vi "RPS Tools.vi"() -> ()   [LabVIEW 2020]
uses:
  Support/Curve fitting data.ctl
panel:
  out "IR Película 2":dbl format="%#.4g"
  out "ángulo B valor medio":dbl
  out "otros ángulos cero":dbl[](array[numeric])
  in  "Stop":bool
  in  "Tab Control":T1(tab)
  in  "Extinction Coefficients TC":dbl[](array[slide]) caption="Extinction Coefficients" step=0.01 scale=-5.0..5.0
  in  "Thicknesses (angstroms) TC":dbl[](array[slide]) caption="Thicknesses (angstroms)" step=5.0 scale=0.0..1000.0 scale format="%#.6g"
  in  "Refractive Indexes TC":dbl[](array[slide]) caption="Refractive Indexes" step=0.01 scale=1.0..5.0 scale format="%#.6g"
  out "q R theoretical TC":dbl caption="qR theoretical" format="%#.5g"
  in  "No.  Layers TC":u32=1 caption="No.  Layers"
  in  "q maximum TC":dbl=89.0 caption="q maximum"
  in  "q minimum TC":dbl=30.0 caption="q minimum"
  in  "l(angstroms) TC":dbl=6328.0 caption="l(angstroms)"
  in  "Resolution TC":dbl=1000.0 caption="Resolution"
  out "SPR Curve":cluster{"EJE X":dbl[], "EJE Y TEÓRICO":dbl[]}(graph)
  in  "No. Layers CF":u32=1 caption="No. Layers"
  in  "l(angstroms) CF":dbl=6328.0 caption="l(angstroms)"
  in  "Losses CF":dbl(slide)=0.9 caption="Losses" step=0.001 scale=0.0..1.0 scale format="%#.6g"
  in  "Error CF":dbl(slide) caption="Error" step=0.01 scale=-5.0..5.0
  in  "Refractive Indexes CF":dbl[](array[slide]) caption="Refractive Indexes" step=0.001 scale=1.0..5.0 scale format="%#.6g"
  in  "Extinction Coefficients CF":dbl[](array[slide]) caption="Extinction Coefficients" step=0.001 scale=-5.0..5.0 scale format="%#.6g"
  in  "Open File":path
  in  "Thicknesses (angstroms) CF":dbl[](array[slide]) caption="Thicknesses (angstroms)" scale=0.0..1000.0 scale format="%#.6g"
  out "CURVE FITTING":T2(graph)
  in  "Load curve":bool
  out "SPR Curve":cluster{"EJE X":dbl[], dbl[]}(graph)
  in  "q Final ECA":dbl caption="q Final"
  in  "q Starting ECA":dbl caption="q Starting"
  in  "Open File ECA":path caption="Open File"
  in  "Realizar Análisis ECA":bool caption="Realizar Análisis"
  out "qR ECA":dbl caption="qR"
  out "Curve width ECA":dbl caption="Curve width" format="%#.3g"
  out "q  Middle ECA":dbl caption="q  Middle"
  out "Minimun Intensity ECA":dbl caption="Minimun Intensity"
  out "Maximum Intensity ECA":dbl caption="Maximum Intensity"
  in  "Calcular ERROR":bool
  out "RI +error BRW":dbl caption="RI +error" format="%#_4g"
  out "qB +error BRW":dbl caption="qB +error"
  in  "Error (degrees) BRW":dbl caption="Error (degrees)"
  out "Refractive Index BRW":dbl caption="Refractive Index" format="%#.4g"
  out "qB BRW":dbl caption="qB"
  in  "Calcular":bool
  in  "q Final BRW":dbl caption="q Final"
  in  "q Starting BRW":dbl caption="q Starting"
  in  "Open File BRW":path caption="Open File"
  out "Curve":cluster{dbl[], dbl[]}(graph)
  out "Curves":cluster{dbl[], dbl[]}[](graph)
  in  "q Final AB":dbl caption="q Final"
  in  "q Starting AB":dbl caption="q Starting"
  in  "Open Film File AB":path caption="Open Film File"
  in  "Open Substrate File AB":path caption="Open Substrate File"
  in  "OK Button":bool
  out "Film RI AB":dbl caption="Film RI" format="%#.4g"
  out "Substrate RI AB":dbl caption="Substrate RI" format="%#.4g"
  out "Substrate qB AB":dbl caption="Substrate qB"
  out "Film qB AB":dbl caption="Film qB"
  in  "calcular error":bool
  in  "Error (degrees) AB":dbl caption="Error (degrees)"
  out "Film qB +error AB":dbl caption="Film qB +error"
  out "Film RI +error AB":dbl caption="Film RI +error" format="%#.4g"
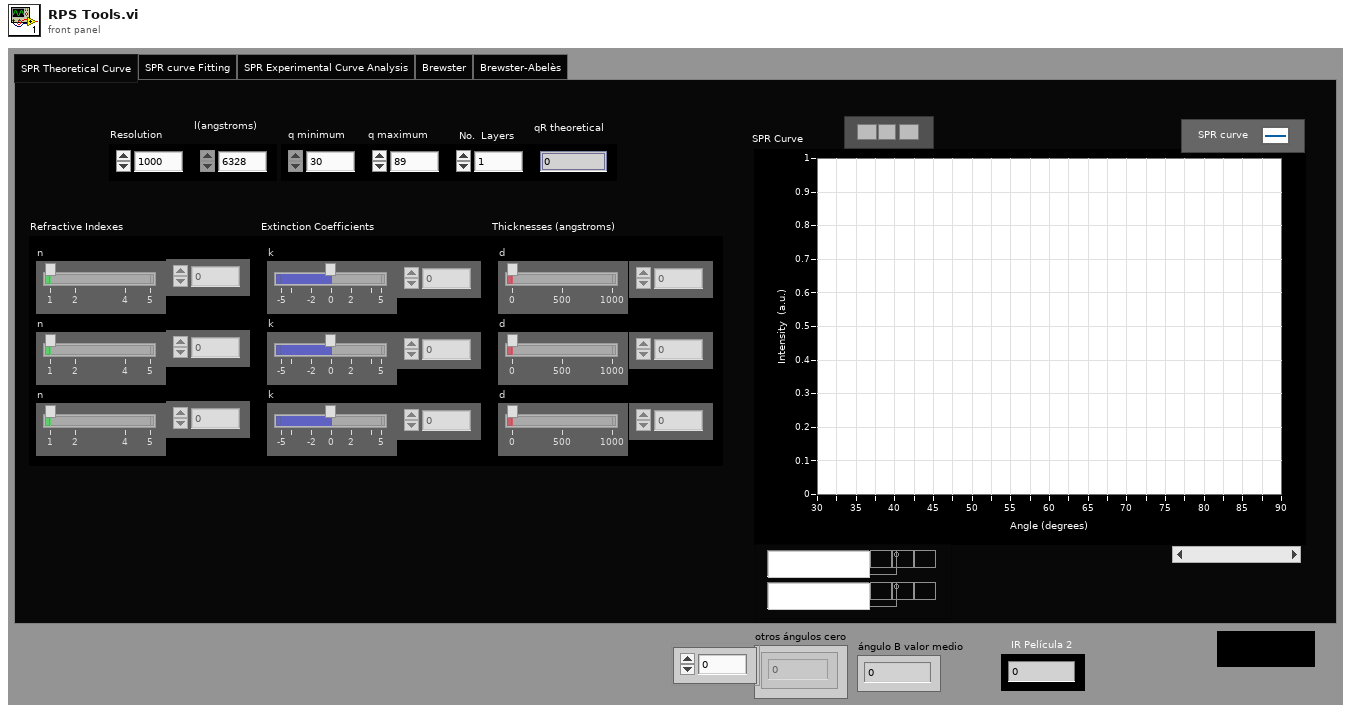
[diagram p1: front panel]
types:
  T1 = enum32{"SPR Theoretical Curve", "SPR curve Fitting", "SPR Experimental Curve Analysis", "Brewster", "Brewster-Abelès"}
  T2 = cluster{"EJE X":dbl[], "EJE Y NORMALIZADO":dbl[]}[]
  T3 = typedef "Curve fitting data.ctl" = cluster{"Número de datos":i32, "EJE X":dbl[], "Ángulo máximo":dbl, "EJE Y":dbl[], "Ángulo mínimo":dbl}
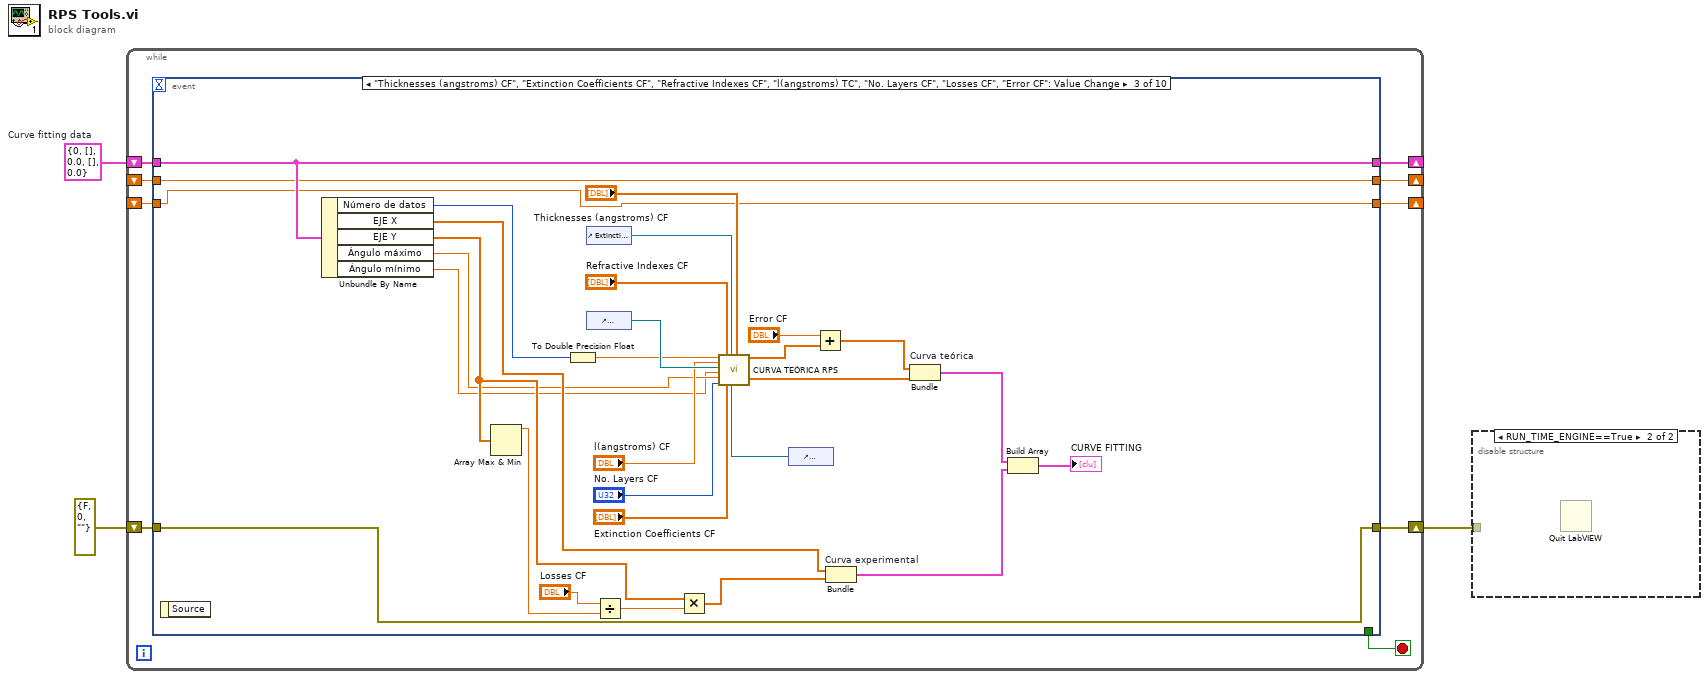
[diagram p0: block diagram]
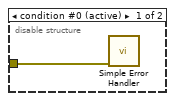
[diagram p2: hidden frame]
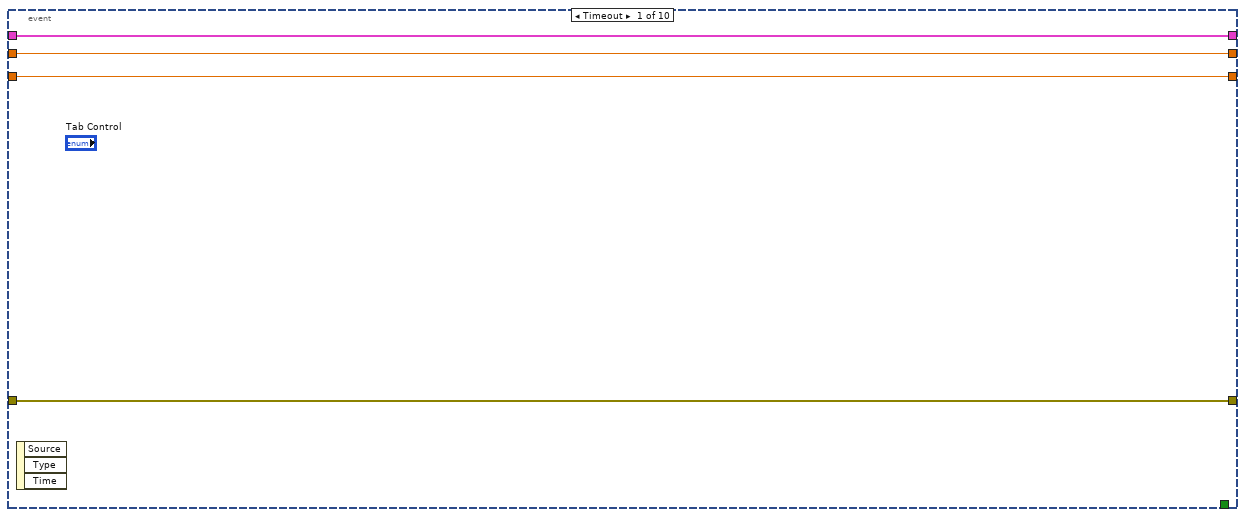
[diagram p3: hidden frame]
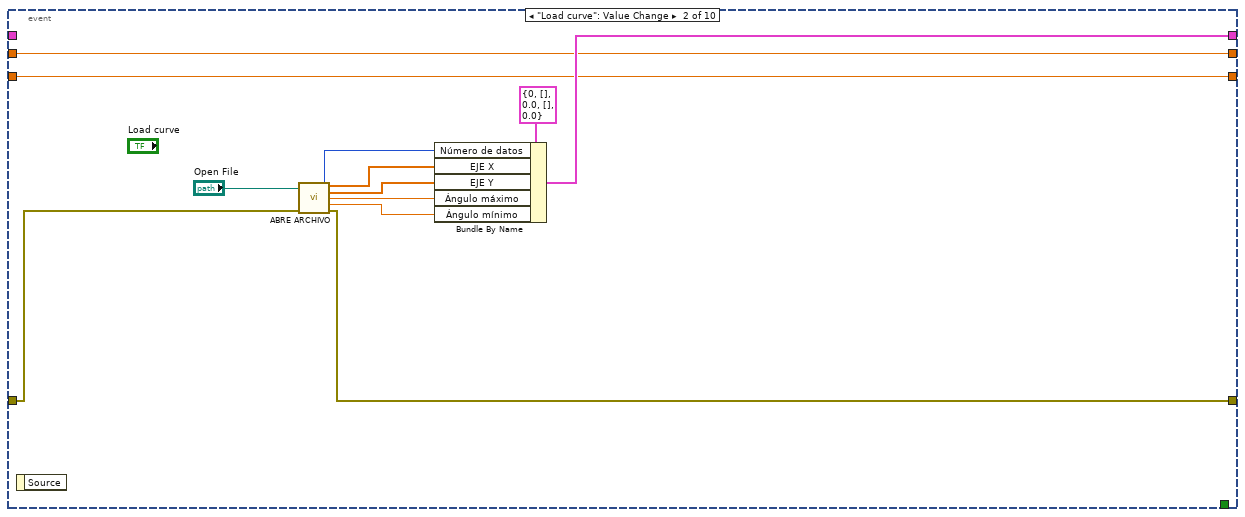
[diagram p4: hidden frame]
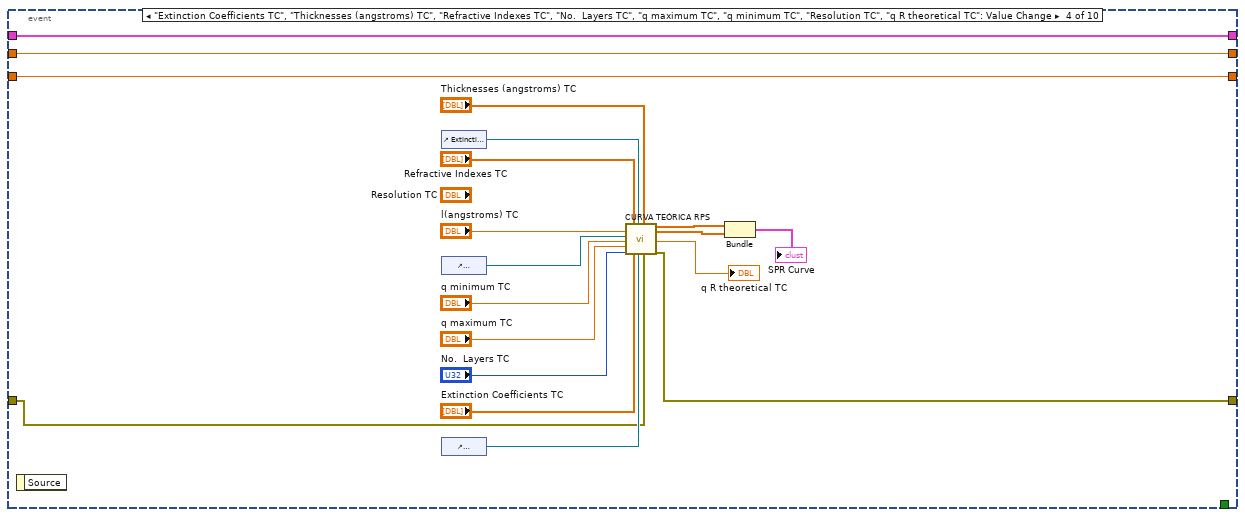
[diagram p5: hidden frame]
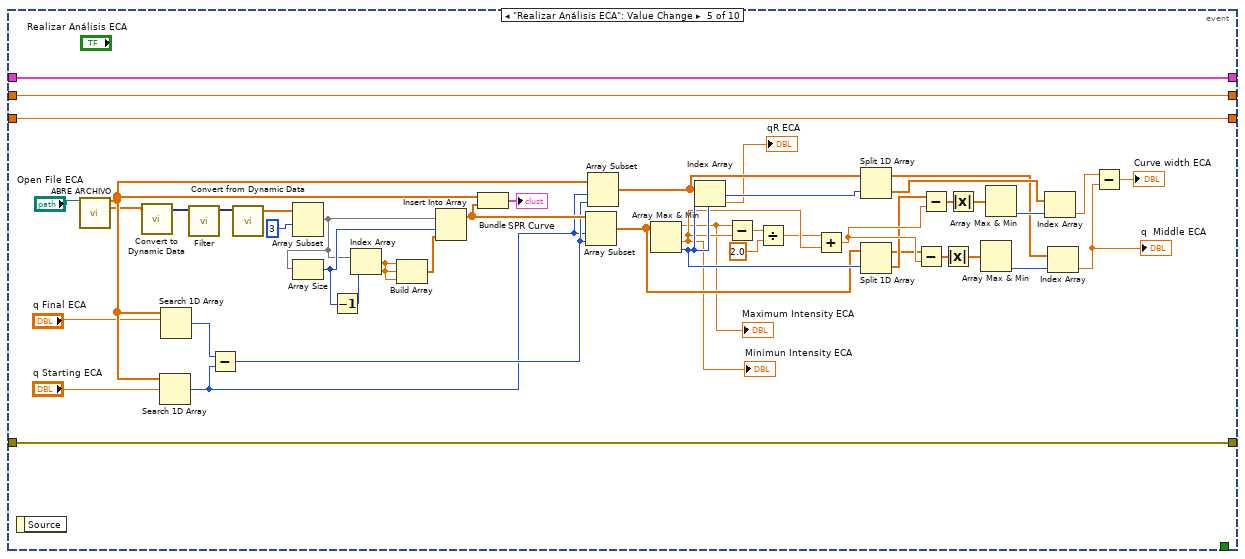
[diagram p6: hidden frame]
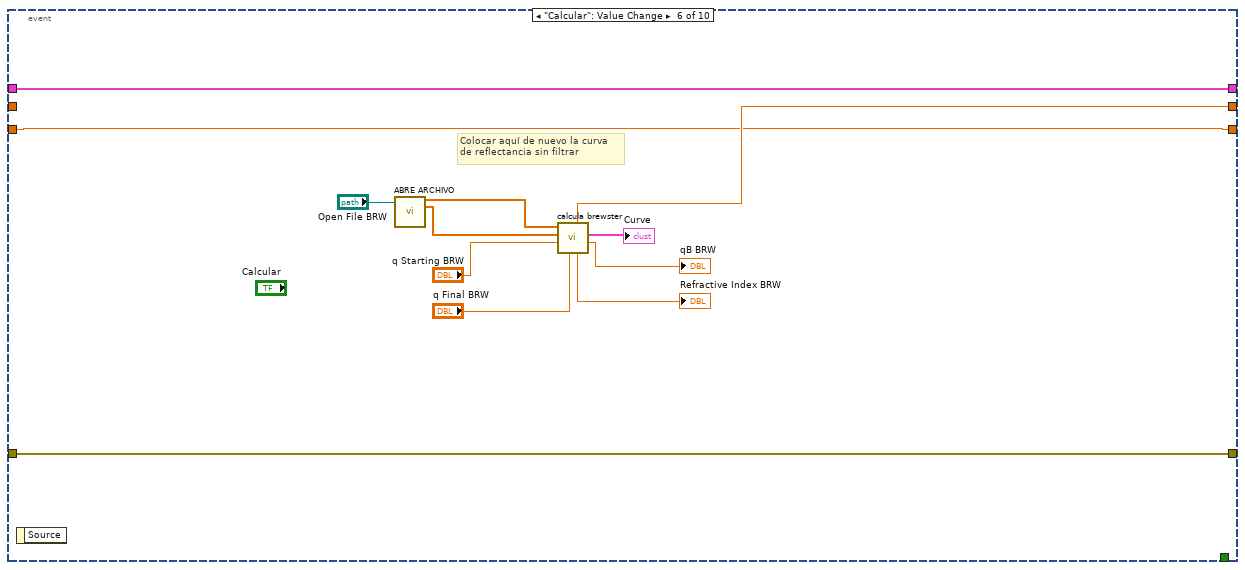
[diagram p7: hidden frame]
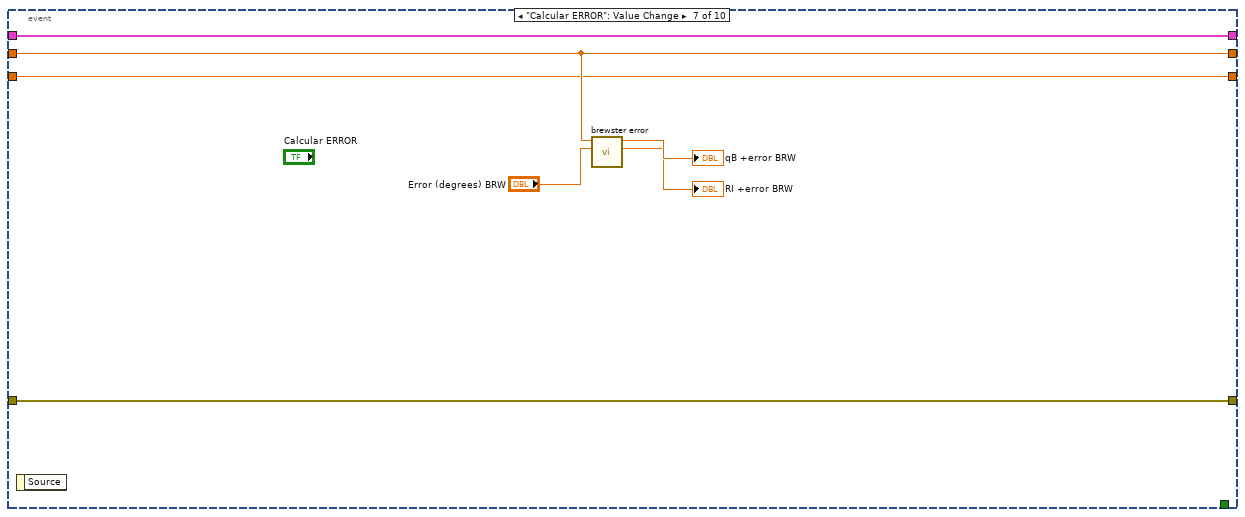
[diagram p8: hidden frame]
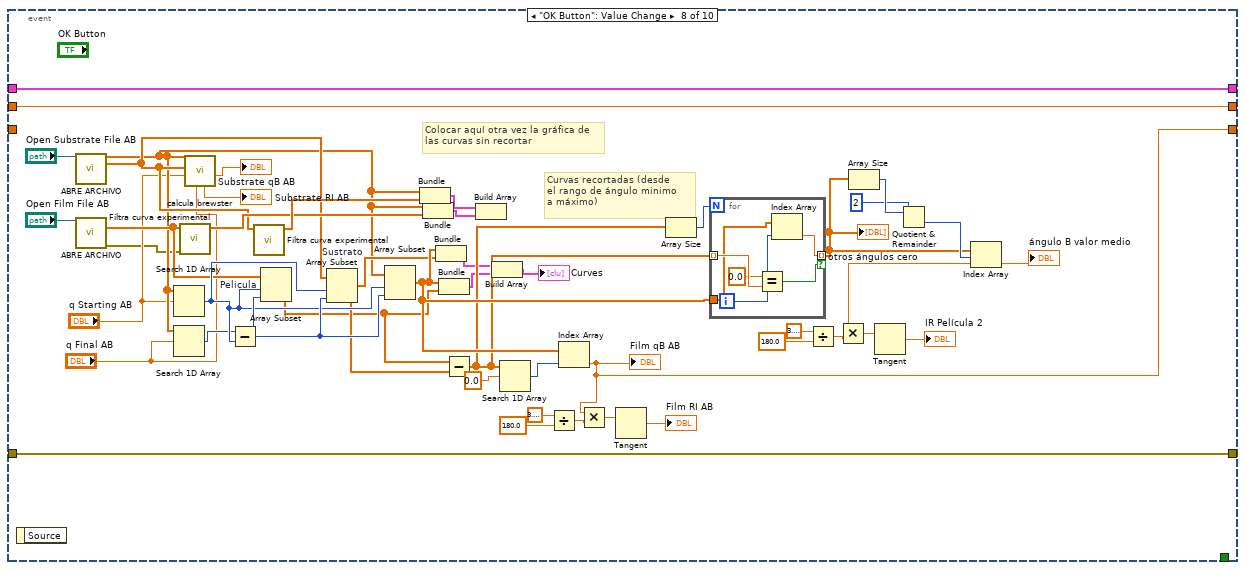
[diagram p9: hidden frame]
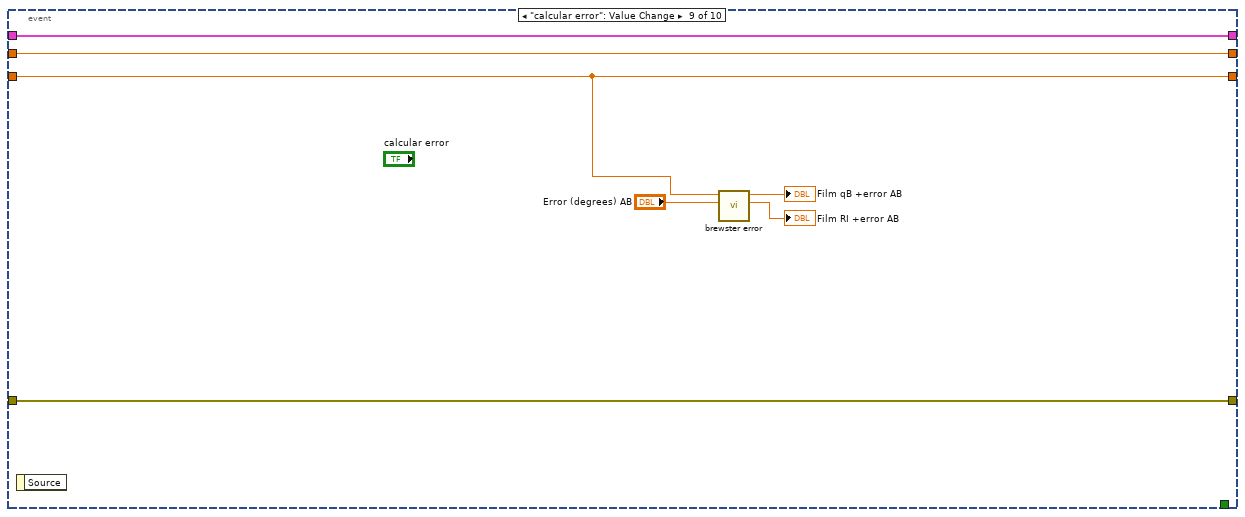
[diagram p10: hidden frame]
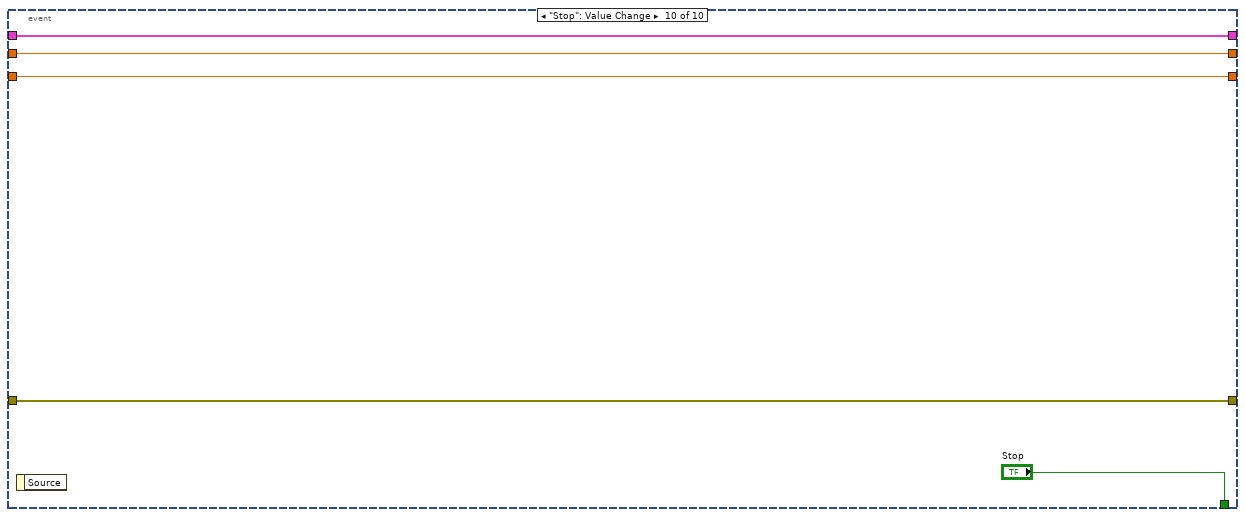
[diagram p11: hidden frame]
diagram:
  w3 = T3 {"Número de datos"=0, "EJE X"=[], "Ángulo máximo"=0.0, "EJE Y"=[], "Ángulo mínimo"=0.0}  # Curve fitting data
  n1 = while {
    shift-right: [w12] -> _
    shift-left: w3 -> [w11]
    shift-right: [w9] -> _
    shift-left: _ -> [w8]
    shift-right: [w7] -> _
    shift-left: _ -> [w6]
    shift-right: [w4] -> w1
    shift-left: errorcluster {"status"=FALSE, "code"=0, "source"=""} ("error constant") -> [w5]
    stop <- w10 stop-if-true
    n2 = event shown="[2] \"Thicknesses (angstroms) CF\", \"Extinction Coefficients CF\", \"Refractive Indexes CF\", \"l(angstroms) TC\", \"No. Layers CF\", \"Losses CF\", \"Error CF\": Value Change" {
      selector: _ -> [_ _ _ _ _ _ _ _ _ _]
      dyn-events: _ -> [_ _ _ _ _ _ _ _ _ _]
      timeout: _ -> [_ _ _ _ _ _ _ _ _ _]
      tunnel: [w16 w21 w37 w76 w122 w134 w141 w187 w200 w205] -> w12
      tunnel: w11 -> [w16 _ w37 w76 w122 w134 w141 w187 w200 w205]
      tunnel: [_ _ _ _ _ _ _ _ _ "Stop"] -> w10
      tunnel: [w15 w20 w31 w61 w79 w125 w140 w186 w199 w203] -> w9
      tunnel: w8 -> [w15 w20 w31 w61 w79 _ w140 w186 w199 w203]
      tunnel: [w14 w19 w30 w60 w78 w124 w136 w143 w198 w202] -> w7
      tunnel: w6 -> [w14 w19 w30 w60 w78 w124 w136 _ w198 w202]
      tunnel: w5 -> [w13 w18 w29 w59 w77 w123 w135 w142 w194 w201]
      tunnel: [w13 w17 w29 w58 w77 w123 w135 w142 w194 w201] -> w4
      event Timeout {
        n3 = event-data() -> ()  [unwired: 1 in, 3 out]
      }
      event "Load curve": Value Change {
        n4 = event-data() -> ()  [unwired: 1 in, 1 out]
        n5 = call "ABRE ARCHIVO.vi"("File Path Control"="Open File", "error in (no error)"=w18) -> ("Número de datos"=w26:i32, "EJE X"=w25:dbl[], "EJE Y"=w24:dbl[], "Ángulo máximo"=w23:dbl, "Ángulo mínimo"=w22:dbl, "error out"=w17:errorcluster)  [unwired: 8 in]
        n6 = Bundle By Name(cluster=T3 {"Número de datos"=0, "EJE X"=[], "Ángulo máximo"=0.0, "EJE Y"=[], "Ángulo mínimo"=0.0} ("Curve data"), "Número de datos"=w26, "EJE X"=w25, "EJE Y"=w24, "Ángulo máximo"=w23, "Ángulo mínimo"=w22) -> (w21:T3)
      }
      event "Thicknesses (angstroms) CF", "Extinction Coefficients CF", "Refractive Indexes CF", "l(angstroms) TC", "No. Layers CF", "Losses CF", "Error CF": Value Change {
        n7 = event-data() -> ()  [unwired: 1 in, 1 out]
        n8 = Unbundle By Name(w37) -> ("Número de datos"=w36:i32, "EJE X"=w35:dbl[], "EJE Y"=w34:dbl[], "Ángulo máximo"=w33:dbl, "Ángulo mínimo"=w32:dbl)
        n9 = Array Max & Min(array=w34) -> (max value=w42:dbl)  [unwired: 3 out]
        n10 = To Double Precision Float(number=w36) -> (double precision float=w50:dbl)
        n11 = control-ref of="Extinction Coefficients CF"() -> (w56:refnum<vi>)
        n12 = control-ref of="Refractive Indexes CF"() -> (w53:refnum<vi>)
        n13 = Divide(x="Losses CF", y=w42) -> (x/y=w43:dbl)
        n14 = Multiply(x=w34, y=w43) -> (x*y=w44:dbl[])
        n15 = control-ref of="Thicknesses (angstroms) CF"() -> (w54:refnum<vi>)
        n16 = call "CURVA TEÓRICA RPS.vi"("Resolución"=w50, "l(angstroms)"="l(angstroms) CF", 2:"Índices de refracción"=w53, "q mínimo"=w32, "q máximo"=w33, "Número de capas"="No. Layers CF", 6:"Índices de refracción"="Refractive Indexes CF", 7:"Coeficientes de extinción"="Extinction Coefficients CF", 8:"Coeficientes de extinción"=w56, "Espesores"=w54, "Espesores (angstroms)"="Thicknesses (angstroms) CF") -> ("EJE X"=w48:dbl[], "EJE Y TEÓRICO"=w49:dbl[])  [unwired: 5 in, 2 out]
        n17 = Add(x="Error CF", y=w48) -> (x+y=w40:dbl[])
        n18 = Bundle "Curva experimental"("EJE X"=w35, w44) -> (w57:cluster{"EJE X":dbl[], dbl[]})  [unwired: 1 in]
        n19 = Bundle "Curva teórica"(w40, "EJE Y TEÓRICO"=w49) -> (w55:cluster{dbl[], "EJE Y TEÓRICO":dbl[]})  [unwired: 1 in]
        n20 = Build Array(w55, w57) -> (→"CURVE FITTING":cluster{"EJE X":dbl[], "EJE Y TEÓRICO":dbl[]}[])
      }
      event "Extinction Coefficients TC", "Thicknesses (angstroms) TC", "Refractive Indexes TC", "No.  Layers TC", "q maximum TC", "q minimum TC", "Resolution TC", "q R theoretical TC": Value Change {
        n21 = event-data() -> ()  [unwired: 1 in, 1 out]
        n22 = control-ref of="Extinction Coefficients TC"() -> (w62:refnum<vi>)
        n23 = control-ref of="Refractive Indexes TC"() -> (w63:refnum<vi>)
        n24 = control-ref of="Thicknesses (angstroms) TC"() -> (w64:refnum<vi>)
        n25 = call "CURVA TEÓRICA RPS.vi"("l(angstroms)"="l(angstroms) TC", 2:"Índices de refracción"=w63, "q mínimo"="q minimum TC", "q máximo"="q maximum TC", "Número de capas"="No.  Layers TC", 6:"Índices de refracción"="Refractive Indexes TC", 7:"Coeficientes de extinción"="Extinction Coefficients TC", 8:"Coeficientes de extinción"=w62, "Espesores"=w64, "Espesores (angstroms)"="Thicknesses (angstroms) TC", "error in (no error)"=w59) -> ("EJE X"=w68:dbl[], "EJE Y TEÓRICO"=w67:dbl[], "q RPS teórico"=→"q R theoretical TC":dbl, "error out"=w58:errorcluster)  [unwired: 5 in]
        n26 = Bundle("EJE X"=w68, "EJE Y TEÓRICO"=w67) -> (→"SPR Curve":cluster{"EJE X":dbl[], "EJE Y TEÓRICO":dbl[]})  [unwired: 1 in]
      }
      event "Realizar Análisis ECA": Value Change {
        n27 = event-data() -> ()  [unwired: 1 in, 1 out]
        n28 = call "ABRE ARCHIVO.vi"("File Path Control"="Open File ECA") -> ("EJE X"=w98:dbl[], "EJE Y"=w88:dbl[])  [unwired: 9 in, 4 out]
        n29 = call "Convert to Dynamic Data"("Array"=w88) -> ("Dynamic Data Type"=w86:dynamicdata)  [unwired: 3 in]
        n30 = Search 1D Array(1D array=w98, element="q Starting ECA") -> (index of element=w95:i32)  [unwired: 1 in]
        n31 = Search 1D Array(1D array=w98, element="q Final ECA") -> (index of element=w85:i32)  [unwired: 1 in]
        n32 = call "Filter"("Signal"=w86) -> ("Filtered Signal"=w87:dynamicdata)  [unwired: 9 in, 1 out]
        n33 = Subtract(x=w85, y=w95) -> (x-y=w96:i32)
        n34 = call "Convert from Dynamic Data"("Dynamic Data Type"=w87) -> ("Array"=w94:dbl[])  [unwired: 3 in]
        n35 = Array Subset(array=w94, index=3 ("length")) -> (w89:dbl[])  [unwired: 1 in]
        n36 = Array Size(array=w89) -> (size(s)=w92:i32)
        n37 = Decrement(x=w92) -> (x-1=w90:i32)
        n38 = Index Array(array=w89, index=w90) -> (element=w91:dbl)
        n39 = Build Array(w91, w91, w91) -> (w93:dbl[])
        n40 = Insert Into Array(array=w89, index=w92, new element=w93) -> (w99:dbl[])
        n41 = Bundle("EJE X"=w98, w99) -> (→"SPR Curve":cluster{"EJE X":dbl[], dbl[]})  [unwired: 1 in]
        n42 = Array Subset(array=w99, index=w95, length=w96) -> (w105:dbl[])
        n43 = Array Subset(array=w98, index=w95, length=w96) -> (w109:dbl[])
        n44 = Array Max & Min(array=w105) -> (max value=w101:dbl, min value=w104:dbl, min index (indices)=w113:i32)  [unwired: 1 out]
        "Minimun Intensity ECA" <- w104
        "Maximum Intensity ECA" <- w101
        n45 = Index Array(array=w109, index=w113) -> (element=→"qR ECA":dbl)
        n46 = Subtract(x=w101, y=w104) -> (x-y=w102:dbl)
        n47 = Divide(x=w102, y=2.0) -> (x/y=w103:dbl)
        n48 = Add(x=w103, y=w104) -> (x+y=w117:dbl)
        n49 = Split 1D Array(array=w109, index=w113) -> (first subarray=w110:dbl[], second subarray=w112:dbl[])
        n50 = Split 1D Array(array=w105, index=w113) -> (first subarray=w106:dbl[], second subarray=w116:dbl[])
        n51 = Subtract(x=w106, y=w117) -> (x-y=w107:dbl[])
        n52 = Subtract(x=w116, y=w117) -> (x-y=w115:dbl[])
        n53 = Absolute Value(x=w107) -> (abs(x)=w108:dbl[])
        n54 = Absolute Value(x=w115) -> (abs(x)=w114:dbl[])
        n55 = Array Max & Min(array=w108) -> (min index (indices)=w111:i32)  [unwired: 3 out]
        n56 = Array Max & Min(array=w114) -> (min index (indices)=w118:i32)  [unwired: 3 out]
        n57 = Index Array(array=w112, index=w118) -> (element=w119:dbl)
        n58 = Index Array(array=w110, index=w111) -> (element=w120:dbl)
        "q  Middle ECA" <- w120
        n59 = Subtract(x=w119, y=w120) -> (x-y=→"Curve width ECA":dbl)
      }
      event "Calcular": Value Change {
        # "Colocar aquí de nuevo la curva\nde reflectancia sin filtrar"
        n60 = event-data() -> ()  [unwired: 1 in, 1 out]
        n61 = call "ABRE ARCHIVO.vi"("File Path Control"="Open File BRW") -> ("EJE X"=w130:dbl[], "EJE Y"=w129:dbl[])  [unwired: 9 in, 4 out]
        n62 = call "calcula brewster.vi"("Ángulo Final"="q Final BRW", "Ángulo Inicial"="q Starting BRW", "EJE Y"=w129, "EJE X"=w130) -> ("Ángulo de Brewster"=→"qB BRW":dbl, "Curva FILTRADA"=→"Curve":cluster{dbl[], dbl[]}, "Índice de Refracción"=→"Refractive Index BRW":dbl, "Numeric Control"=w125:dbl)  [unwired: 3 in, 1 out]
      }
      event "Calcular ERROR": Value Change {
        n63 = event-data() -> ()  [unwired: 1 in, 1 out]
        n64 = call "brewster error.vi"("Error (grados)"="Error (degrees) BRW", "Numeric Control"=w140) -> ("Índice de Refracción +error"=→"RI +error BRW":dbl, "Ángulo de Brewster +error"=→"qB +error BRW":dbl)  [unwired: 8 in]
      }
      event "OK Button": Value Change {
        # "Curvas recortadas (desde\nel rango de ángulo minimo \na máximo)"
        # "Colocar aquí otra vez la gráfica de\nlas curvas sin recortar"
        n65 = event-data() -> ()  [unwired: 1 in, 1 out]
        n66 = call "ABRE ARCHIVO.vi"("File Path Control"="Open Substrate File AB") -> ("EJE X"=w166:dbl[], "EJE Y"=w168:dbl[])  [unwired: 9 in, 4 out]
        n67 = call "ABRE ARCHIVO.vi"("File Path Control"="Open Film File AB") -> ("EJE Y"=w167:dbl[], "error out"=w154:errorcluster)  [unwired: 9 in, 4 out]
        n68 = Search 1D Array(1D array=w166, element="q Starting AB") -> (index of element=w174:i32)  [unwired: 1 in]
        n69 = Search 1D Array(1D array=w166, element="q Final AB") -> (index of element=w157:i32)  [unwired: 1 in]
        n70 = call "Filtra curva experimental.vi"("error in (no error)"=w154, "Y"=w167) -> ("Y Filtrada"=w176:dbl[])  [unwired: 7 in, 2 out]
        n71 = call "calcula brewster.vi"("Ángulo Final"="q Final AB", "Ángulo Inicial"="q Starting AB", "EJE Y"=w168, "EJE X"=w166) -> ("Ángulo de Brewster"=→"Substrate qB AB":dbl, "Índice de Refracción"=→"Substrate RI AB":dbl)  [unwired: 3 in, 3 out]
        n72 = Subtract(x=w157, y=w174) -> (x-y=w175:i32)
        n73 = call "Filtra curva experimental.vi"("Y"=w168) -> ("Y Filtrada"=w177:dbl[])  [unwired: 8 in, 2 out]
        n74 = Array Subset "Pelicula"(array=w167, index=w174, length=w175) -> (w169:dbl[])
        n75 = Array Subset "Sustrato"(array=w168, index=w174, length=w175) -> (w170:dbl[])
        n76 = Array Subset(array=w166, index=w174, length=w175) -> (w178:dbl[])
        n77 = Bundle("EJE X"=w166, "Y Filtrada"=w177) -> (w161:cluster{"EJE X":dbl[], "Y Filtrada":dbl[]})  [unwired: 1 in]
        n78 = Bundle("EJE X"=w166, "Y Filtrada"=w176) -> (w160:cluster{"EJE X":dbl[], "Y Filtrada":dbl[]})  [unwired: 1 in]
        n79 = Bundle(w178, w170) -> (w171:cluster{dbl[], dbl[]})  [unwired: 1 in]
        n80 = Bundle(w178, w169) -> (w158:cluster{dbl[], dbl[]})  [unwired: 1 in]
        n81 = Subtract(x=w169, y=w170) -> (x-y=w173:dbl[])
        n82 = Build Array(w161, w160) -> ()  [unwired: 1 out]
        n83 = Build Array(w171, w158) -> (→"Curves":cluster{dbl[], dbl[]}[])
        n84 = Search 1D Array(1D array=w173, element=0.0) -> (index of element=w162:i32)  [unwired: 1 in]
        n85 = Divide(x=3.141592653589793, y=180.0) -> (x/y=w165:dbl)
        n86 = Index Array(array=w178, index=w162) -> (element=w143:dbl)
        "Film qB AB" <- w143
        n87 = Multiply(x=w143, y=w165) -> (x*y=w164:dbl)
        n88 = Tangent(1:w164) -> (0:→"Film RI AB":dbl)
        n89 = Array Size(array=w173) -> (size(s)=w172:i32)
        n90 = for {
          N: w172 -> [_]
          tunnel: w173 -> [w193] mode=indexing
          tunnel: [w188] -> w180 mode=indexing if=w191
          tunnel: w178 -> [w190]
          i -> [w189]
          n91 = Equal?(x=0.0, y=w193) -> (x = y?=w191:bool)
          n92 = Index Array(array=w190, index=w189) -> (element=w188:dbl)
        }
        "otros ángulos cero" <- w180
        n93 = Divide(x=3.141592653589793, y=180.0) -> (x/y=w181:dbl)
        n94 = Array Size(array=w180) -> (size(s)=w179:i32)
        n95 = Quotient & Remainder(x=w179, y=2) -> (floor(x/y)=w185:i32)  [unwired: 1 out]
        n96 = Index Array(array=w180, index=w185) -> (element=w182:dbl)
        "ángulo B valor medio" <- w182
        n97 = Multiply(x=w182, y=w181) -> (x*y=w184:dbl)
        n98 = Tangent(1:w184) -> (0:→"IR Película 2":dbl)
      }
      event "calcular error": Value Change {
        n99 = event-data() -> ()  [unwired: 1 in, 1 out]
        n100 = call "brewster error.vi"("Error (grados)"="Error (degrees) AB", "Numeric Control"=w198) -> ("Índice de Refracción +error"=→"Film RI +error AB":dbl, "Ángulo de Brewster +error"=→"Film qB +error AB":dbl)  [unwired: 8 in]
      }
      event "Stop": Value Change {
        n101 = event-data() -> ()  [unwired: 1 in, 1 out]
      }
    }
  }
  n102 = disable-structure shown="RUN_TIME_ENGINE==True" {
    disable-tunnel: w1 -> [w206 _]
    frame condition #0 (active) {
      n103 = call <vilib>:"Simple Error Handler.vi"("error in (no error)"=w206) -> ()  [unwired: 4 in, 5 out]
    }
    frame condition #1 {
      n104 = Quit LabVIEW() -> ()  [unwired: 1 in]
    }
  }
